vi "Add Library To Project.vi"(6 "Template Library Name":string, 8 "error in":errorcluster, 9 "Library Path":path, 10 "Project:Active Project":refnum<vi>) -> (0 "error out":errorcluster)   [LabVIEW 2021, in "_Template.lvlib" / "_Template.lvclass"]
uses:
  _Template.lvclass
  _Template.lvclass/_Template.ctl
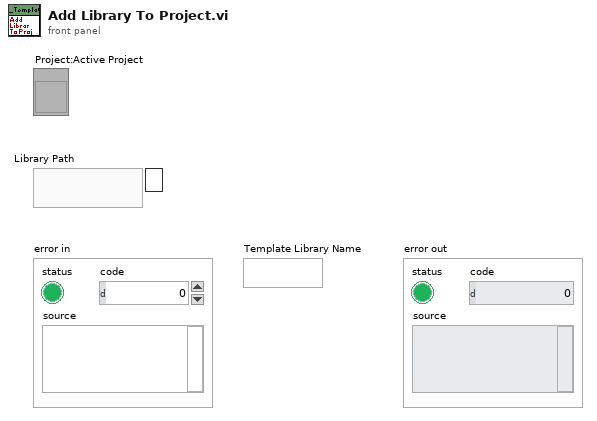
[diagram p1: front panel]
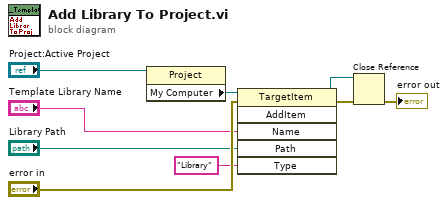
[diagram p0: block diagram]
diagram:
  n1 = property class="Project"(reference="Project:Active Project") -> ("My Computer"=w8:refnum<vi>)  [unwired: 1 in, 2 out]
  n2 = invoke class="TargetItem" method="AddItem"(reference=w8, error in="error in", "Name"="Template Library Name", "Path"="Library Path", "Type"="Library") -> (reference out=w4:refnum<vi>, error out=w3:errorcluster)  [unwired: 1 in, 4 out]
  n3 = Close Reference(reference=w4, error in (no error)=w3) -> (error out=→"error out":errorcluster)
